vi "XGT 개별읽기 Enquire.vi"(5 "명령어타입":string="SS", 7 "명령어":string="R", 9 "블록 변수":cluster{"변수길이":string, "변수이름":string}[](array[cluster])=[{"변수길이"="06", "변수이름"="%MW020"}, {"변수길이"="06", "변수이름"="%PW001"}], 10 "블록수":string="02", 11 "국번":string="01") -> (3 "연속연결 Enquire문":string)   [LabVIEW 2014]
panel:
  in  "Header":string="\u0005"
  in  "BCC":string
  in  "Tail":string="\u0004"
  # "국번 1의 M020 번지에서 1Word, \n     P001번지에서 1Word를 읽음"
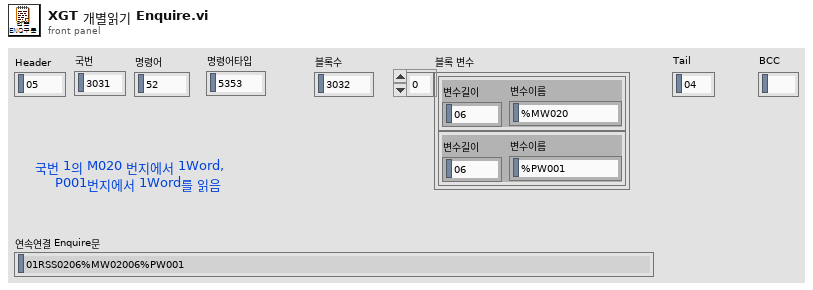
[diagram p1: front panel]
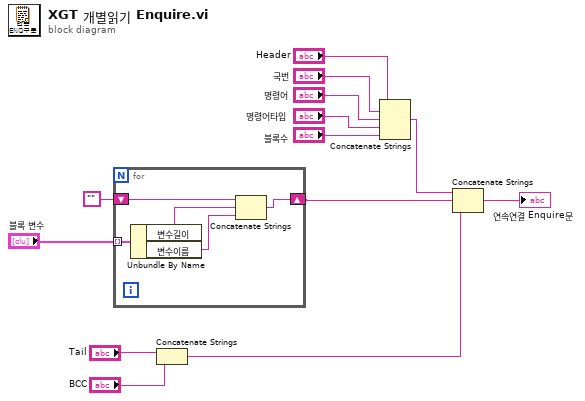
[diagram p0: block diagram]
diagram:
  n1 = for {
    tunnel: "블록 변수" -> [w18] mode=indexing
    shift-right: [w14] -> w3
    shift-left: "" -> [w17]
    n2 = Unbundle By Name(w18) -> ("변수길이"=w16:string, "변수이름"=w15:string)
    n3 = Concatenate Strings(w17, w16, w15) -> (w14:string)
  }
  n4 = Concatenate Strings("Tail", "BCC") -> (w2:string)
  n5 = Concatenate Strings("Header", "국번", "명령어", "명령어타입", "블록수") -> (w4:string)
  n6 = Concatenate Strings(w4, w3, w2) -> (→"연속연결 Enquire문":string)
